vi "Set Camera.vi"(8 "error in (no error)":errorcluster, 10 "Camera":T1, 11 "FormulaG API in":refnum<class "FormulaG API.lvclass">) -> (0 "error out":errorcluster, 3 "FormulaG API out":refnum<class "FormulaG API.lvclass">)   [LabVIEW 2020, in "FormulaG.lvlib" / "FormulaG API.lvclass"]
uses:
  FormulaG API.lvclass
  FormulaLV-Common/Camera.ctl
  Command.ctl
  FormulaG API.lvclass/FormulaG API.ctl
  <vilib>/IlluminatedG/lv-stream/stream/Stream.lvclass/Stream.ctl
  <vilib>/IlluminatedG/lv-stream/stream/Dispatch Sniffer Data.vi
  <vilib>/IlluminatedG/lv-stream/stream/Prepared.vi
  <vilib>/IlluminatedG/lv-stream/Endpoint/Cast Sniffer Callback.vi
  <vilib>/IlluminatedG/IG WebSocket Stream/Stream-Websocket/WebsocketStream/WebsocketStream.lvclass
  C:/Program Files (x86)/National Instruments/LabVIEW 2020/vi.lib/IlluminatedG/lv-stream/stream/Stream.lvclass
  <vilib>/Utility/error.llb/Error Cluster From Error Code.vi
  <vilib>/IlluminatedG/lv-stream/stream/Stream.lvclass
  FormulaLV-Common/FormulaG-Common.lvlib
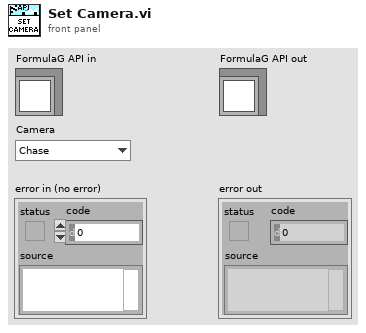
[diagram p1: front panel]
types:
  T1 = typedef "FormulaG-Common.lvlib/Camera.ctl" = enum16{"Chase", "Overhead"}
  T2 = enum16{"big-endian, network order", "native, host order", "little-endian"}
  T3 = typedef "FormulaG.lvlib/FormulaG API.lvclass/Command.ctl" = enum8{"None", "Reset Car", "Request Ranges", "Control Car", "Request Info", "Set Options", "Set Camera", "Set Pause"}
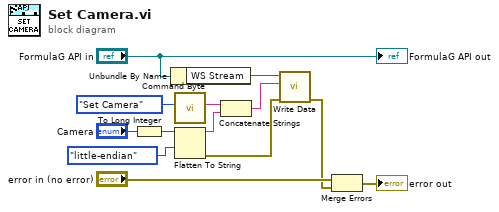
[diagram p0: block diagram]
diagram:
  n1 = To Long Integer(number="Camera") -> (32bit integer=w6:i32)
  n2 = Unbundle By Name("FormulaG API in") -> ("WS Stream"=w9:refnum<class "WebsocketStream.lvclass">)
  n3 = call "Command Byte.vi"("Command"=Command."Set Camera") -> ("Command Byte"=w10:string)  [unwired: 10 in]
  n4 = Flatten To String(anything=w6, byte order (0:big-endian, network order)=T2."little-endian") -> (data string=w4:string, error out=w3:errorcluster)  [unwired: 2 in, 1 out]
  n5 = Concatenate Strings(w10, w4) -> (w8:string)
  n6 = call <vilib>:"Write Data.vi"("error in (no error)"=w3, "Data"=w8, "Stream in"=w9) -> ("error out"=w1:errorcluster)  [unwired: 7 in, 1 out]
  n7 = Merge Errors("error in (no error)", w1) -> (→"error out":errorcluster)
  "FormulaG API out" <- "FormulaG API in"
